vi "PhotonPoseEstimator_PackConfig.vi"(0 "FallBack Strategy":T2, 1 "BaseNTName":string="/photonvision", 4 "Initial Pose":T9={"Translation3d"={"X"=0.0, "Y"=0.0, "Z"=0.0}, "Rotation3d"={"Q_quaternion"={"R"=1.0, "V"=[0.0, 0.0, 0.0]}}} {"Translation3d"."Z" format="%14.3f"; "Translation3d"."Y" format="%14.3f"; "Translation3d"."X" format="%14.3f"}, 5 "Custom AprilTag Field":T7={"AprilTagMap"={}, "FieldLength"=0.0, "FieldWidth"=0.0, "OriginPosition "=enum."kBlueAllianceWallRightSide,", "OriginPose3d"={"Translation3d"={"X"=0.0, "Y"=0.0, "Z"=0.0}, "Rotation3d"={"Q_quaternion"={"R"=1.0, "V"=[0.0, 0.0, 0.0]}}}} {"OriginPose3d"."Translation3d"."Z" format="%14.3f"; "OriginPose3d"."Translation3d"."Y" format="%14.3f"; "OriginPose3d"."Translation3d"."X" format="%14.3f"}, 6 "RobotToCamera":T3={"TRANSLATION3D"={"X"=0.0, "Y"=0.0, "Z"=0.0}, "ROTATION3D"={"Q_quaternion"={"R"=1.0, "V"=[0.0, 0.0, 0.0]}}, "XF"=FALSE} {"TRANSLATION3D"."Z" format="%14.3f"; "TRANSLATION3D"."Y" format="%14.3f"; "TRANSLATION3D"."X" format="%14.3f"}, 7 "Use Custom Field":bool, 8 "HighestAmbiguity":dbl=10.0, 9 "PirmaryStrategy":T2, 10 "Camera":string="HD_USB_Camera", 11 "AprilTagField":T1(ring)=enum."2024 Crescendo") -> (3 "PoseEstimator_Configuration":T11)   [LabVIEW 2019, in "PhotonVisionLib.lvlib"]
doc: "Provided data from polling a camera, update the estimated position of the robot. Returns empty if there are no cameras set or no targets were found from the cameras. \n\nNOTE: The inputs are only used on the first call. After that changes to the inputs are ignored. If anyone wants any of these items to be dynamic, please submit an enhancement request through github\n\nInputs:\n - BaseTNName -- string - Base network tables name. Default: /photonvision\n - CustomAprilTagField -- cluster -- If a custom field is used, this defines the field.\n - UseCustomField -- boolean -- use a custom apriltag field instead of one of the predefined ones.\n - AprilTagField -- enum - Field selector\n - Camera -- string - Camera name\n - Primary Strategy -- enum - Primary estimation strategy\n - HighestAmbiguity -- double -- Highest permitted ambiguity value\n - RobotToCamera -- Transform3d -- Position of camera on robot\n - InitialPose -- Pose3d - Initial location of robot on the field.\n - Fallback Strategy -- enum - Strategy to use when primary strategy fails.\n\nOutputs:\n -- PhotonPoseEstimator _Configuration -- data cluster -- Pose Estimator Configuration data"
uses:
  PhotonVisionLib.lvlib
  Enum/PhotonPoseStrategy_ENUM.ctl
  <vilib>/Rock Robotics/WPI/ThirdParty/JAS_Junk/TrajLib/TypeDef/POSE3D.ctl
  <vilib>/Rock Robotics/WPI/ThirdParty/JAS_Junk/TrajLib/TypeDef/TRANSLATION3D.ctl
  <vilib>/Rock Robotics/WPI/ThirdParty/JAS_Junk/TrajLib/TypeDef/ROTATION3D.ctl
  <vilib>/Rock Robotics/WPI/ThirdParty/JAS_Junk/TrajLib/TypeDef/QUATERNION.ctl
  Ref/PhotonPoseEstimator_Configuration_REF.ctl
  TypeDef/PhotonPoseEstimator_Configuration.ctl
  <vilib>/Rock Robotics/WPI/ThirdParty/JAS_Junk/TrajLib/TypeDef/AprilTagFieldLayout.ctl
  <vilib>/Rock Robotics/WPI/ThirdParty/JAS_Junk/TrajLib/TypeDef/AprilTag.ctl
  <vilib>/Rock Robotics/WPI/ThirdParty/JAS_Junk/TrajLib/Enum/AprilTagFieldLayoutOrignPosition_ENUM.ctl
  <vilib>/Rock Robotics/WPI/ThirdParty/JAS_Junk/TrajLib/TypeDef/TRANSFORM3D.ctl
  <vilib>/Rock Robotics/WPI/ThirdParty/JAS_Junk/TrajLib/Trajectory_Library.lvlib
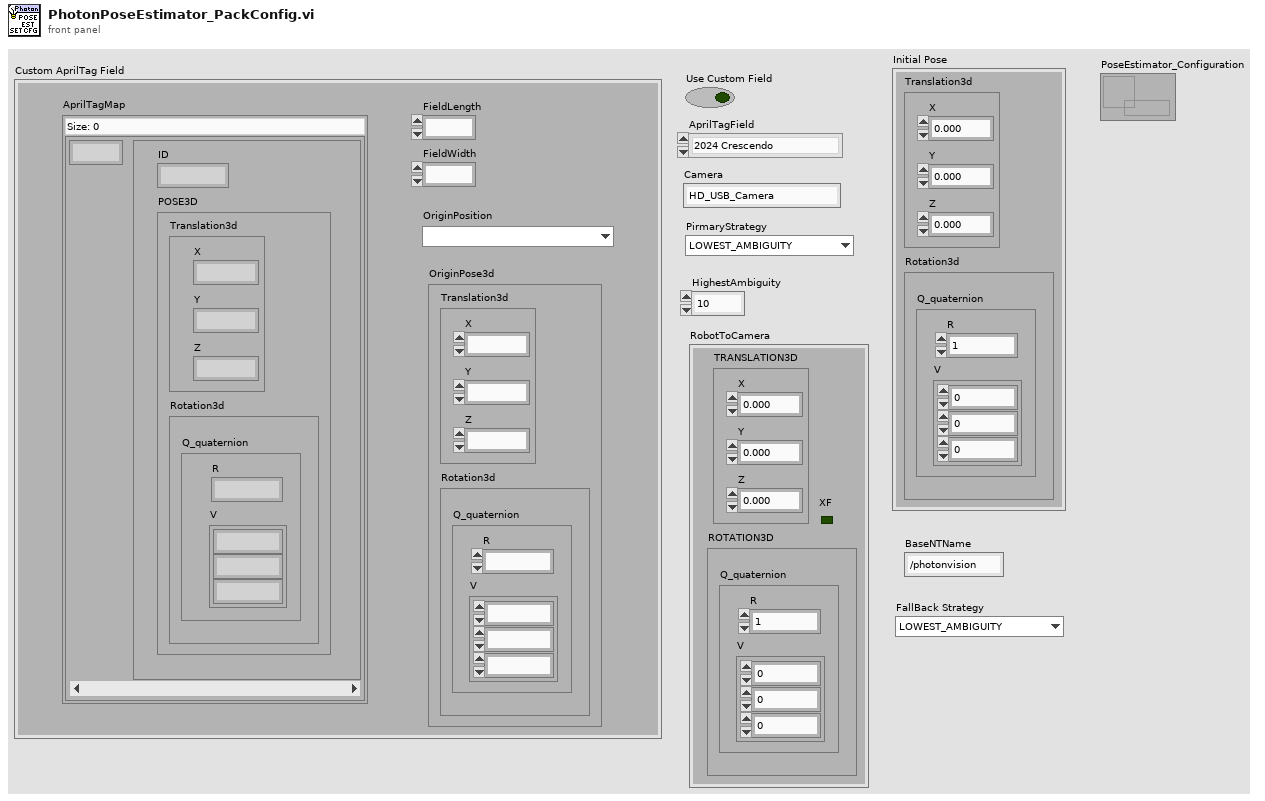
[diagram p1: front panel]
types:
  T1 = enum16{"2022 Rapid React", "2023 Charged Up", "2024 Crescendo"}
  T2 = typedef "PhotonVisionLib.lvlib/PhotonPoseStrategy_ENUM.ctl" = enum16{"LOWEST_AMBIGUITY", "CLOSEST_TO_CAMERA_HEIGHT", "CLOSEST_TO_REFERENCE_POSE", "CLOSEST_TO_LAST_POSE", "AVERAGE_BEST_TARGETS", "MULTI_TAG_PNP_ON_COPROCESSOR", "MULTI_TAG_PNP_ON_RIO"}
  T3 = typedef "Trajectory_Library.lvlib/TRANSFORM3D.ctl" = cluster{"TRANSLATION3D":T4, "ROTATION3D":T5, "XF":bool}
  T4 = typedef "Trajectory_Library.lvlib/TRANSLATION3D.ctl" = cluster{"X":dbl, "Y":dbl, "Z":dbl}
  T5 = typedef "Trajectory_Library.lvlib/ROTATION3D.ctl" = cluster{"Q_quaternion":T6}
  T6 = typedef "Trajectory_Library.lvlib/QUATERNION.ctl" = cluster{"R":dbl, "V":dbl[]}
  T7 = typedef "Trajectory_Library.lvlib/AprilTagFieldLayout.ctl" = cluster{"AprilTagMap":map{i32, T8}, "FieldLength":dbl, "FieldWidth":dbl, "OriginPosition ":T10, "OriginPose3d":T9}
  T8 = typedef "Trajectory_Library.lvlib/AprilTag.ctl" = cluster{"ID":i32, "POSE3D":T9}
  T9 = typedef "Trajectory_Library.lvlib/POSE3D.ctl" = cluster{"Translation3d":T4, "Rotation3d":T5}
  T10 = typedef "Trajectory_Library.lvlib/AprilTagFieldLayoutOrignPosition_ENUM.ctl" = enum16{"kBlueAllianceWallRightSide,", "kRedAllianceWallRightSide,"}
  T11 = typedef "PhotonVisionLib.lvlib/PhotonPoseEstimator_Configuration_REF.ctl" = refnum<data-value>
  T12 = typedef "PhotonVisionLib.lvlib/PhotonPoseEstimator_Configuration.ctl" = cluster{"Primary Strategy":T2, "Camera":string, "Initial Pose":T9, "HighestAmbiguity":dbl, "Use Custom Field":bool, "Custom AprilTag Field":T7, "RobotToCamera":T3, "FallBack Strategy":T2, "BaseNTName":string, "AprilTagField":enum16{"2022 Rapid React", "2023 Charged Up", "2024 Crescendo"}}
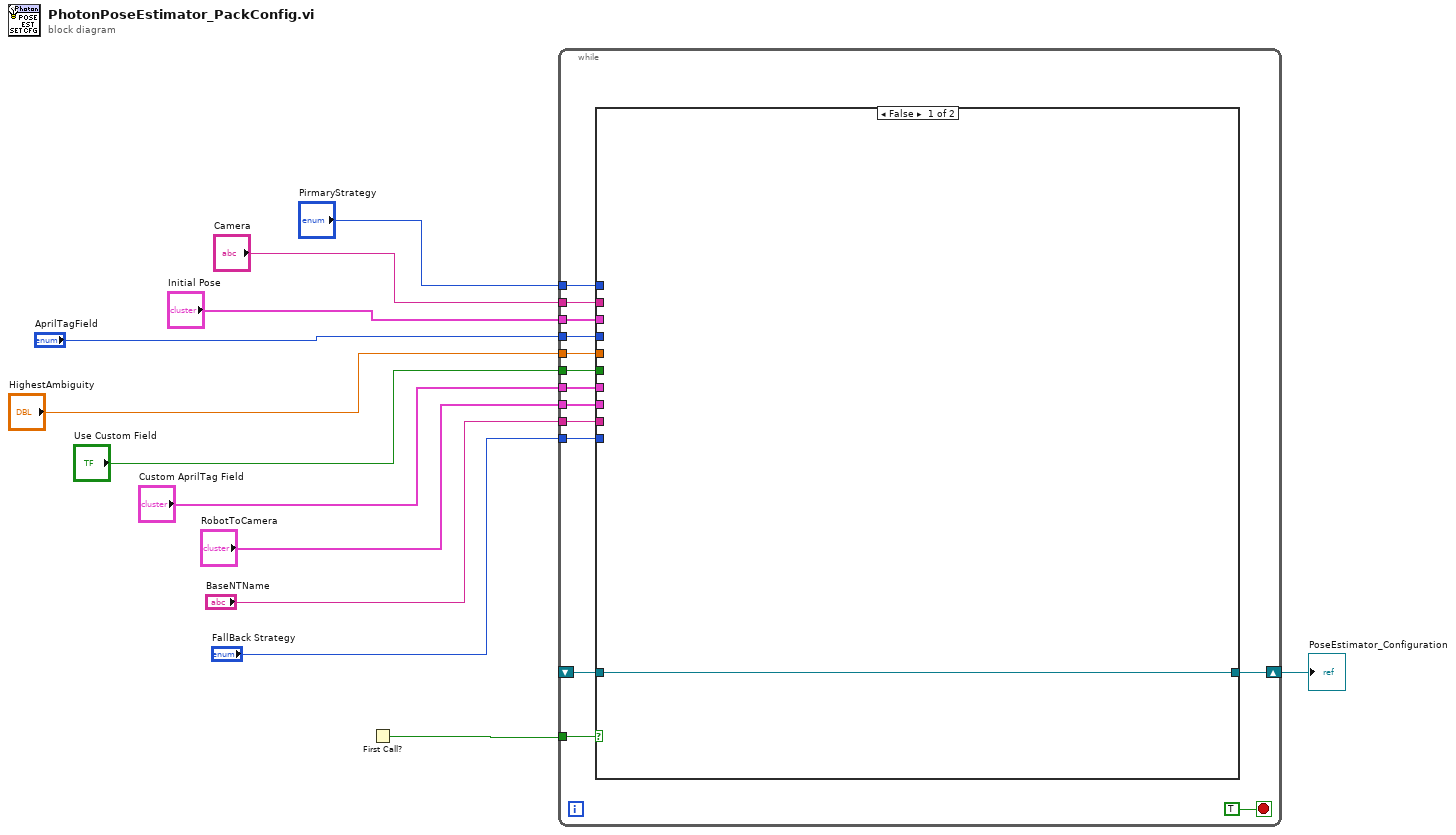
[diagram p0: block diagram]
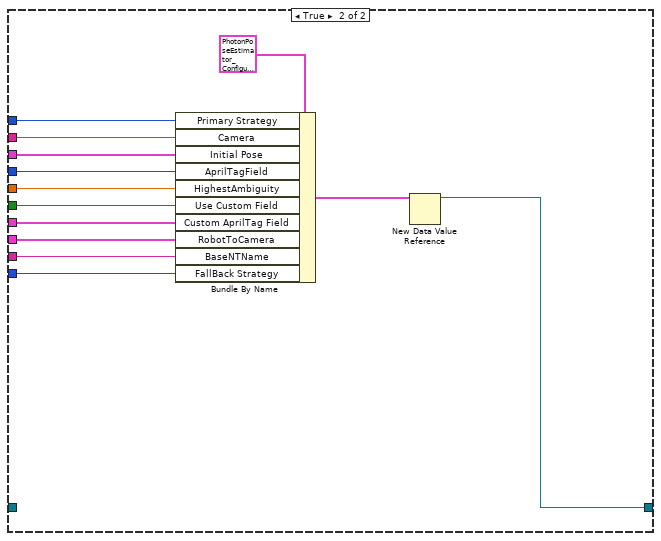
[diagram p2: hidden frame]
diagram:
  n1 = First Call?() -> (First Call?: T/F=w1:bool)
  n2 = while {
    tunnel: "PirmaryStrategy" -> [w26]
    tunnel: "Camera" -> [w25]
    tunnel: "Initial Pose" -> [w24]
    tunnel: "HighestAmbiguity" -> [w23]
    tunnel: "Use Custom Field" -> [w22]
    tunnel: "Custom AprilTag Field" -> [w21]
    tunnel: "RobotToCamera" -> [w20]
    tunnel: "BaseNTName" -> [w19]
    tunnel: "FallBack Strategy" -> [w18]
    tunnel: "AprilTagField" -> [w17]
    tunnel: w1 -> [w15]
    shift-right: [w16] -> w2
    shift-left: _ -> [w13]
    stop <- TRUE stop-if-true
    n3 = case shown="False" w15 {
      tunnel: w26 -> [_ w39]
      tunnel: w25 -> [_ w38]
      tunnel: w24 -> [_ w37]
      tunnel: w23 -> [_ w36]
      tunnel: w22 -> [_ w35]
      tunnel: w21 -> [_ w34]
      tunnel: w20 -> [_ w33]
      tunnel: w19 -> [_ w32]
      tunnel: w18 -> [_ w31]
      tunnel: w17 -> [_ w30]
      tunnel: [w27 w28] -> w16
      tunnel: w13 -> [w27 _]
      frame False {
      }
      frame True {
        n4 = Bundle By Name(cluster=T12 {"Primary Strategy"=enum."LOWEST_AMBIGUITY", "Camera"="", "Initial Pose"={"Translation3d"={"X"=0.0, "Y"=0.0, "Z"=0.0}, "Rotation3d"={"Q_quaternion"={"R"=1.0, "V"=[0.0, 0.0, 0.0]}}}, "HighestAmbiguity"=0.0, "Use Custom Field"=FALSE, "Custom AprilTag Field"={"AprilTagMap"={}, "FieldLength"=0.0, "FieldWidth"=0.0, "OriginPosition "=enum."kBlueAllianceWallRightSide,", "OriginPose3d"={"Translation3d"={"X"=0.0, "Y"=0.0, "Z"=0.0}, "Rotation3d"={"Q_quaternion"={"R"=1.0, "V"=[0.0, 0.0, 0.0]}}}}, "RobotToCamera"={"TRANSLATION3D"={"X"=0.0, "Y"=0.0, "Z"=0.0}, "ROTATION3D"={"Q_quaternion"={"R"=1.0, "V"=[0.0, 0.0, 0.0]}}, "XF"=FALSE}, "FallBack Strategy"=enum."LOWEST_AMBIGUITY", "BaseNTName"="/photonvision", "AprilTagField"=enum."2022 Rapid React"} ("Configuration"), "Primary Strategy"=w39, "Camera"=w38, "Initial Pose"=w37, "AprilTagField"=w30, "HighestAmbiguity"=w36, "Use Custom Field"=w35, "Custom AprilTag Field"=w34, "RobotToCamera"=w33, "BaseNTName"=w32, "FallBack Strategy"=w31) -> (w29:T12)
        n5 = New Data Value Reference(data value=w29) -> (data value reference=w28:refnum<data-value>)  [unwired: 1 in, 1 out]
      }
    }
  }
  "PoseEstimator_Configuration" <- w2
